vi "Append Front Panel Image.vi"(0 "PDF Report IN":refnum<class "PDF Report Class.lvclass">, 1 "Scale (%)":sgl=100.0, 3 "Border":T1={"Show?"=FALSE, "Thickness (point)"=0.5, "Color"=0}, 5 "VI reference":refnum<vi>, 9 "visible area only? (T)":bool=TRUE, 11 "error in (no error)":errorcluster, 12 "Caption":string, 14 "Position and indentation":T2={"Alignment"=enum."Center", "X "=0.0, "Y"=0.0, "Indentation"=0.0}) -> (4 "PDF Report OUT":refnum<class "PDF Report Class.lvclass">, 15 "error out":errorcluster)   [LabVIEW 2019]
doc: "Creates an image of the front panel of the VI you specify in <B>VI reference</B> and appends it to a PDF report.\n\n<B>FRANÇAIS</B>\nCréation de l'image du panneau avant spécifié par <B>VI reference</B> et ajout au rapport PDF.\n\nVersion 1.0\nDeveloped by Jean-Marc Simard\nCopyright © 2010, Exaprom Inc.\nAll rights reserved.\nLicense: BSD\n\nWith iTextSharp 4.1.6 (http://itextsharp.sourceforge.net)\nunder Mozilla Public License Version 1.1\n(http://www.mozilla.org/MPL/MPL-1.1.html)"
uses:
  <userlib>/Exaprom PDF/LV Class/PDF Report Class/PDF Report Class.lvclass
  <userlib>/Exaprom PDF/Controls/Image Controls/Image alignment and position.ctl
  <userlib>/Exaprom PDF/Controls/Image Controls/Image aligment.ctl
  <userlib>/Exaprom PDF/Controls/Image Controls/Image border.ctl
  C:/Program Files/National Instruments/LabVIEW 2019/user.lib/Exaprom PDF/DLL/itextsharp.dll
  DLL/itextsharp.dll
panel:
  out "Size (points)":cluster{"TotalHeight":sgl, "TotalWidth":sgl}
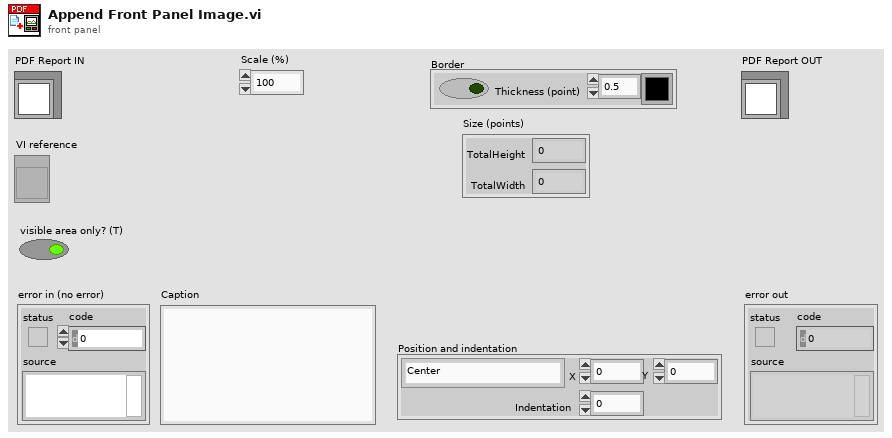
[diagram p1: front panel]
types:
  T1 = typedef "Image border.ctl" = cluster{"Show?":bool, "Thickness (point)":sgl, "Color":u32}
  T2 = typedef "Image alignment and position.ctl" = cluster{"Alignment":T3, "X ":sgl, "Y":sgl, "Indentation":sgl}
  T3 = typedef "Image aligment.ctl" = enum16{"Absolute (X,Y)", "Left", "Center", "Right", "Left (textwrap)", "Right (textwrap)"}
  T4 = typedef "imagedata.ctl" = cluster{"image type":i32, "image depth":i32, "image":u8[], "mask":u8[], "colors":u32[], "Rectangle":cluster{"left":i16, "top":i16, "right":i16, "bottom":i16}}
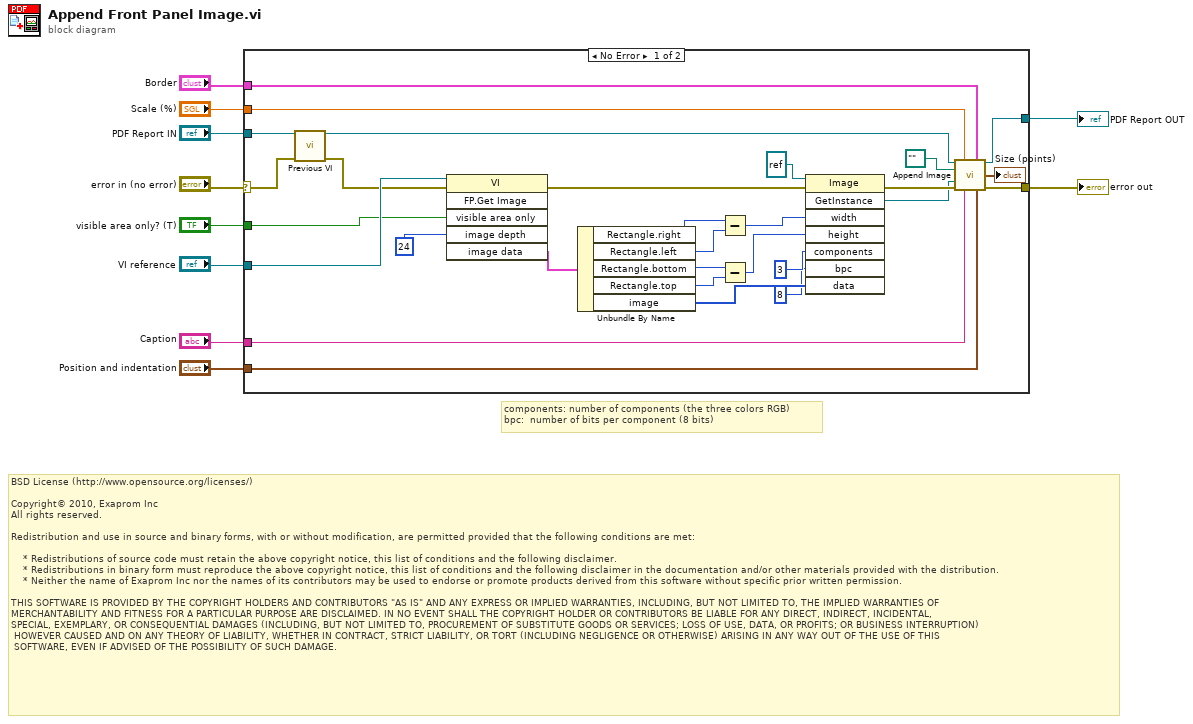
[diagram p0: block diagram]
diagram:
  # "components: number of components (the three colors RGB)\nbpc:  number of bits per component (8 bits)"
  # "BSD License (http://www.opensource.org/licenses/)\n\nCopyright© 2010, Exaprom Inc\nAll rights reserved.\n\nRedistribution and use in source and binary forms, with or without modification, are permitted provided that the following conditions are met:\n\n    * Redistributions of source code must retain the above copyright notice, this list of conditions and the following disclaimer.\n    * Redistributions in binary form must reproduce the above copyright notice, this list of conditions and the following disclaimer in the documentation and/or other materials provided with the distribution.\n    * Neither the name of Exaprom Inc nor the names of its contributors may be used to endorse or promote products derived from this software without specific prior written permission.\n\nTHIS SOFTWARE IS PROVIDED BY THE COPYRIGHT HOLDERS AND CONTRIBUTORS \"AS IS\" AND ANY EXPRESS OR IMPLIED WARRANTIES, INCLUDING, BUT NOT LIMITED TO, THE IMPLIED WARRANTIES OF \nMERCHANTABILITY AND FITNESS FOR A PARTICULAR PURPOSE ARE DISCLAIMED. IN NO EVENT SHALL THE COPYRIGHT HOLDER OR CONTRIBUTORS BE LIABLE FOR ANY DIRECT, INDIRECT, INCIDENTAL,\nSPECIAL, EXEMPLARY, OR CONSEQUENTIAL DAMAGES (INCLUDING, BUT NOT LIMITED TO, PROCUREMENT OF SUBSTITUTE GOODS OR SERVICES; LOSS OF USE, DATA, OR PROFITS; OR BUSINESS INTERRUPTION)\n HOWEVER CAUSED AND ON ANY THEORY OF LIABILITY, WHETHER IN CONTRACT, STRICT LIABILITY, OR TORT (INCLUDING NEGLIGENCE OR OTHERWISE) ARISING IN ANY WAY OUT OF THE USE OF THIS\n SOFTWARE, EVEN IF ADVISED OF THE POSSIBILITY OF SUCH DAMAGE."
  n1 = case shown="No Error" "error in (no error)" {
    selector: "error in (no error)" -> [w12 w41]
    tunnel: [w22 w41] -> w2
    tunnel: "VI reference" -> [w38 _]
    tunnel: [w34 w40] -> w1
    tunnel: "PDF Report IN" -> [w35 w40]
    tunnel: "Caption" -> [w21 _]
    tunnel: "Position and indentation" -> [w20 _]
    tunnel: "Border" -> [w19 _]
    tunnel: "Scale (%)" -> [w18 _]
    tunnel: "visible area only? (T)" -> [w16 _]
    frame No Error {
      n2 = call <userlib>:"Previous VI.vi"("PDF Report IN"=w35, "error in (no error)"=w12) -> ("PDF Report OUT"=w13:refnum<class "PDF Report Class.lvclass">, "error out"=w11:errorcluster)  [unwired: 12 out]
      n3 = invoke class="VI" method="FP.Get Image"(reference=w38, error in=w11, "visible area only"=w16, "image depth"=24 ("Image Depth")) -> (error out=w39:errorcluster, "image data"=w33:T4)  [unwired: 2 in, 4 out]
      n4 = Unbundle By Name(w33) -> ("Rectangle.right"=w31:i16, "Rectangle.left"=w30:i16, "Rectangle.bottom"=w28:i16, "Rectangle.top"=w27:i16, "image"=w24:u8[])
      n5 = Subtract(x=w31, y=w30) -> (x-y=w29:i16)
      n6 = Subtract(x=w28, y=w27) -> (x-y=w26:i16)
      n7 = invoke class="Image" method="GetInstance"(reference=refnum<k24> refnum ("image"), error in=w39, "width"=w29, "height"=w26, "components"=3, "bpc"=8, "data"=w24) -> (error out=w36:errorcluster, "GetInstance"=w15:refnum<k24>)  [unwired: 1 in, 6 out]
      n8 = call <userlib>:"Append Image.vi"("PDF Report IN"=w13, "Scale (%)"=w18, "Border"=w19, "Image path"=path "" ("path"), "Image Ref iTexSharp"=w15, "error in (no error)"=w36, "Caption"=w21, "Position and indentation"=w20) -> ("PDF Report OUT"=w34:refnum<class "PDF Report Class.lvclass">, "Size (points)"=→"Size (points)":cluster{"TotalHeight":sgl, "TotalWidth":sgl}, "error out"=w22:errorcluster)  [unwired: 5 out]
    }
    frame Error {
    }
  }
  "error out" <- w2
  "PDF Report OUT" <- w1
